vi "minimal_acquire.vi"(8 "error in (no error)":errorcluster, 11 "Hamamatsu_C9100-13 in":refnum<class "Hamamatsu_C9100-13.lvclass">) -> (0 "error out":errorcluster, 3 "Hamamatsu_C9100-13 out":refnum<class "Hamamatsu_C9100-13.lvclass">)   [LabVIEW 2013, in "Hamamatsu_C9100-13.lvclass"]
uses:
  Hamamatsu_C9100-13.lvclass
  Hamamatsu_C9100-13.lvclass/Hamamatsu_C9100-13.ctl
  Experiment/Globals.vi
panel:
  out "Camera Temperature":dbl
  out "Last Valid Buffer Index":i32
  out "Acquiring?":bool
  out "Last Valid Buffer Number":i32
  out "Buffer Number":i32
  out "x-y":i32
  out "New Data?":bool
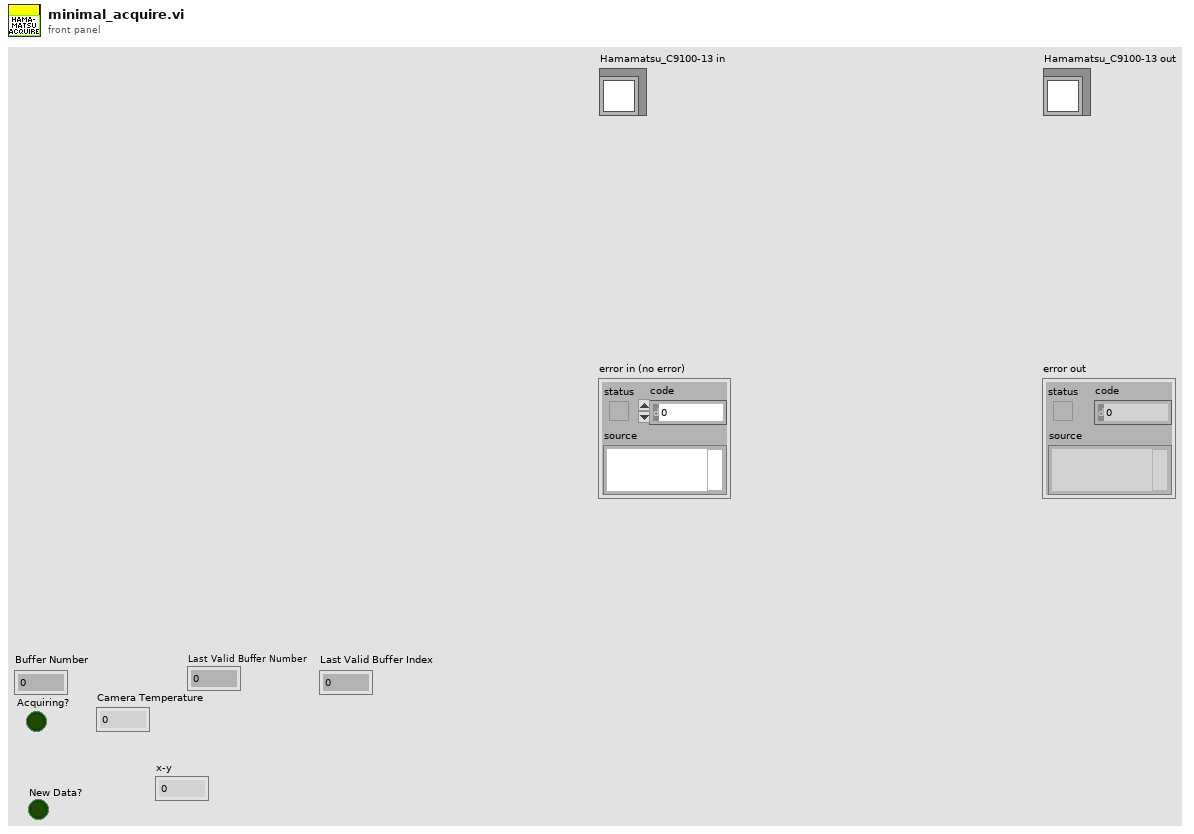
[diagram p1: front panel]
types:
  T1 = typedef "IMAQ Image.ctl" = refnum<image>
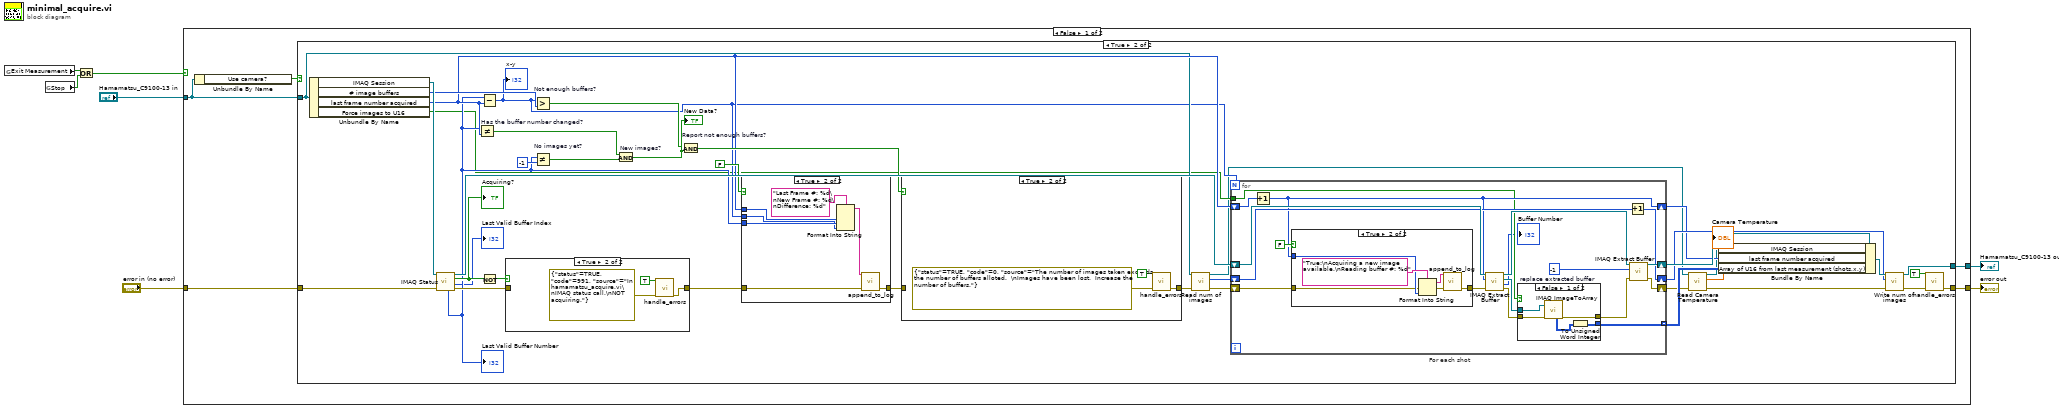
[diagram p0: block diagram]
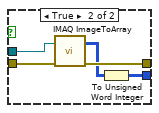
[diagram p5: hidden frame]
diagram:
  n1 = global read "Globals.vi" "Exit Measurement"() -> (w5:bool)
  n2 = global read "Globals.vi" "Stop"() -> (w4:bool)
  n3 = Or(x=w5, y=w4) -> (x .or. y?=w3:bool)
  n4 = case shown="False" w3 {
    tunnel: [w12 w105] -> w1
    tunnel: [w9 w106] -> w6
    tunnel: "Hamamatsu_C9100-13 in" -> [w10 w106]
    tunnel: "error in (no error)" -> [w8 w105]
    frame False {
      n5 = Unbundle By Name(w10) -> ("Use camera?"=w11:bool)
      n6 = case shown="True" w11 {
        tunnel: w8 -> [w14 w45]
        tunnel: [w14 w24] -> w12
        tunnel: w10 -> [w13 w29]
        tunnel: [w13 w30] -> w9
        frame False {
        }
        frame True {
          n7 = Unbundle By Name(w29) -> ("IMAQ Session"=w44:refnum<k11>, "# image buffers"=w43:i32, "last frame number acquired"=w32:i32, "Force images to U16"=w22:bool)
          n8 = call <vilib>:"IMAQ Status.vi"("error in (no error)"=w45, "IMAQ Session In"=w44) -> ("error out"=w35:errorcluster, "Last Valid Buffer Index"=→"Last Valid Buffer Index":i32, "Acquiring?"=w46:bool, "IMAQ Session Out"=w52:refnum<k11>, "Last Valid Buffer Number"=w31:i32)  [unwired: 5 in]
          "Last Valid Buffer Number" <- w31
          "Acquiring?" <- w46
          n9 = Not Equal? "Has the buffer number changed?"(x=w31, y=w32) -> (x != y?=w48:bool)
          n10 = Subtract(x=w31, y=w32) -> (x-y=w26:i32)
          "x-y" <- w26
          n11 = Not(x=w46) -> (.not. x?=w36:bool)
          n12 = case shown="True" w36 {
            tunnel: [w62 w65] -> w33
            tunnel: w35 -> [w62 _]
            frame False {
            }
            frame True {
              n13 = call "handle_errors.vi"("Exit Operation"=TRUE, "error in (no error)"=errorcluster {"status"=TRUE, "code"=991, "source"="In hamamatsu_acquire.vi\nIMAQ status call.\nNOT acquiring."} ("error constant")) -> ("error out"=w65:errorcluster)  [unwired: 13 in]
            }
          }
          n14 = Greater? "Not enough buffers?"(x=w26, y=w43) -> (0:w50:bool)
          n15 = Not Equal? "No images yet?"(x=w31, y=-1) -> (x != y?=w47:bool)
          n16 = Compound Arithmetic op=AND "New images?"(w48, w47) -> (w53:bool)
          "New Data?" <- w53
          n17 = And "Report not enough buffers?"(x=w50, y=w53) -> (x .and. y?=w49:bool)
          n18 = case shown="True" FALSE ("Enable") {
            tunnel: [w54 w61] -> w16
            tunnel: w33 -> [w54 w60]
            tunnel: w32 -> [_ w57]
            tunnel: w31 -> [_ w56]
            tunnel: w26 -> [_ w55]
            frame False {
            }
            frame True {
              n19 = Format Into String(format string="Last Frame #: %d\nNew Frame #: %d\nDifference: %d", w57, w56, w55) -> (resulting string=w58:string)  [unwired: 2 in, 1 out]
              n20 = call "append_to_log.vi"("error in"=w60, "string"=w58) -> ("error out"=w61:errorcluster)  [unwired: 9 in]
            }
          }
          n21 = case shown="True" w49 {
            tunnel: w16 -> [w101 _]
            tunnel: [w101 w104] -> w28
            frame False {
            }
            frame True {
              n22 = call "handle_errors.vi"("Exit Operation"=TRUE ("Exit Measurement"), "error in (no error)"=errorcluster {"status"=TRUE, "code"=0, "source"="The number of images taken exceeds the number of buffers alloted.  \nImages have been lost.  Increase the number of buffers."} ("error constant")) -> ("error out"=w104:errorcluster)  [unwired: 13 in]
            }
          }
          n23 = call-dynamic "Read num of images.vi"("error in (no error)"=w28, "Camera in"=w29) -> ("error out"=w37:errorcluster, "# of images"=w38:u32, "Camera out"=w18:refnum<class "Hamamatsu_C9100-13.lvclass">)  [unwired: 7 in]
          n24 = for "For each shot" {
            N: w26 -> [_]
            shift-right: [w75] -> w39
            shift-left: w32 -> [w83]
            shift-right: [w80] -> w42
            shift-left: w52 -> [w82]
            shift-right: [w77] -> w20
            shift-left: w37 -> [w74]
            shift-right: [w78] -> w40
            shift-left: w38 -> [w79]
            tunnel: [w68] -> w27 mode=indexing
            tunnel: w22 -> [w69]
            w66 = -1  # replace extracted buffer
            n25 = Increment(x=w83) -> (x+1=w75:i32)
            n26 = case shown="True" FALSE ("Enable") {
              tunnel: w74 -> [w94 w98]
              tunnel: [w94 w95] -> w73
              tunnel: w75 -> [_ w99]
              frame False {
              }
              frame True {
                n27 = Format Into String(format string="True:\nAcquiring a new image available.\nReading buffer #: %d", error in=w98, w99) -> (resulting string=w97:string, error out=w96:errorcluster)  [unwired: 1 in]
                n28 = call "append_to_log.vi"("error in"=w96, "string"=w97) -> ("error out"=w95:errorcluster)  [unwired: 9 in]
              }
            }
            n29 = call <vilib>:"IMAQ Extract Buffer.vi"("error in (no error)"=w73, "Buffer to extract"=w75, "IMAQ Session In"=w82) -> ("error out"=w72:errorcluster, "Buffer Number"=→"Buffer Number":i32, "Image Out"=w70:T1, "IMAQ Session Out"=w81:refnum<k11>)  [unwired: 3 in, 2 out]
            n30 = case shown="False" w69 {
              tunnel: w72 -> [w88 w93]
              tunnel: [w87 w92] -> w71
              tunnel: [w84 w91] -> w68
              tunnel: w70 -> [w86 w89]
              frame False {
                n31 = call "IMAQ ImageToArray"("error in (no error)"=w88, "Image"=w86) -> ("Image Pixels (U16)"=w85:u16[][], "error out"=w87:errorcluster)  [unwired: 2 in, 3 out]
                n32 = To Unsigned Word Integer(number=w85) -> (unsigned 16bit integer=w84:u16[][])
              }
              frame True {
                n33 = call "IMAQ ImageToArray"("error in (no error)"=w93, "Image"=w89) -> ("error out"=w92:errorcluster, "Image Pixels (I16)"=w90:i16[][])  [unwired: 2 in, 3 out]
                n34 = To Unsigned Word Integer(number=w90) -> (unsigned 16bit integer=w91:u16[][])
              }
            }
            n35 = Increment(x=w79) -> (x+1=w78:u32)
            n36 = call <vilib>:"IMAQ Extract Buffer.vi"("error in (no error)"=w71, "Buffer to extract"=w66, "IMAQ Session In"=w81) -> ("error out"=w77:errorcluster, "IMAQ Session Out"=w80:refnum<k11>)  [unwired: 3 in, 4 out]
          }
          n37 = call-dynamic "Read Camera Temperature.vi"("error in (no error)"=w20, "Hamamatsu_C9100-13 in"=w18) -> ("error out"=w19:errorcluster, "Camera Temperature"=→"Camera Temperature":dbl, "Hamamatsu_C9100-13 out"=w17:refnum<class "Hamamatsu_C9100-13.lvclass">)  [unwired: 7 in]
          n38 = Bundle By Name(cluster=w17, "IMAQ Session"=w42, "last frame number acquired"=w39, "Array of U16 from last measurement (shots,x,y)"=w27) -> (w41:refnum<class "Hamamatsu_C9100-13.lvclass">)
          n39 = call-dynamic "Write num of images.vi"("error in (no error)"=w19, "# of images"=w40, "Camera in"=w41) -> ("error out"=w25:errorcluster, "Camera out"=w30:refnum<class "Hamamatsu_C9100-13.lvclass">)  [unwired: 7 in]
          n40 = call "handle_errors.vi"("Exit Operation"=TRUE ("Exit Measurement"), "error in (no error)"=w25) -> ("error out"=w24:errorcluster)  [unwired: 13 in]
        }
      }
    }
    frame True {
    }
  }
  "error out" <- w1
  "Hamamatsu_C9100-13 out" <- w6
